vi "channelNames2SortedArray.vi"(10 "DAQmx \nPhysical Channel":tag="Dev2/ai0:31") -> (2 "names out":string[](array[string]))   [LabVIEW 2017]
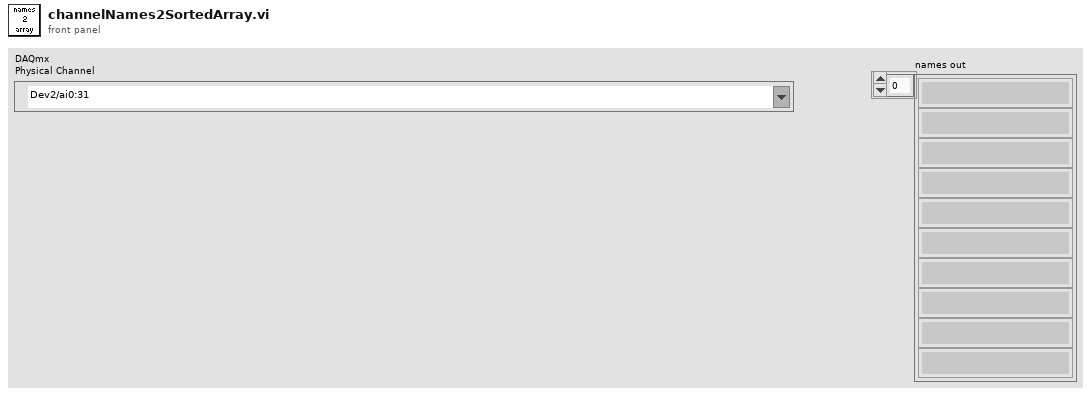
[diagram p1: front panel]
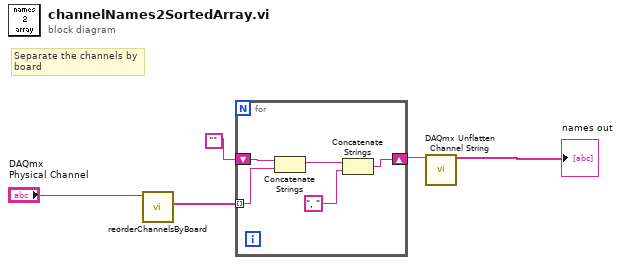
[diagram p0: block diagram]
diagram:
  # "Separate the channels by\nboard"
  n1 = call "reorderChannelsByBoard.vi"("DAQmx \nPhysical Channel"="DAQmx \nPhysical Channel") -> ("Separated inputs\nas strings"=w4:string[])  [unwired: 8 in, 2 out]
  n2 = for {
    tunnel: w4 -> [w9] mode=indexing
    shift-right: [w8] -> w2
    shift-left: "" -> [w10]
    n3 = Concatenate Strings(w10, w9) -> (w7:string)
    n4 = Concatenate Strings(w7, ", ") -> (w8:string)
  }
  n5 = call <vilib>:"DAQmx Unflatten Channel String.vi"("names in"=w2) -> ("names out"=→"names out":string[])  [unwired: 13 in, 1 out]
